vi "ObjectCacher(VariantInterface).vi"(8 "Enum(Get)":T1=enum."Get", 9 "type-postfix":string, 10 "Variant":variant, 11 "key":string[](array[string])) -> (1 "found/Replace":bool[](array[boolean]), 2 "names":string[](array[string]), 3 "values":variant[](array[variant]), 4 "cacher":variant)   [LabVIEW 2017]
uses:
  ObjectCacher-Operation.ctl
  <userlib>/_OpenG.lib/md5/md5.llb/MD5 Message Digest (Hexadecimal String)__ogtk.vi
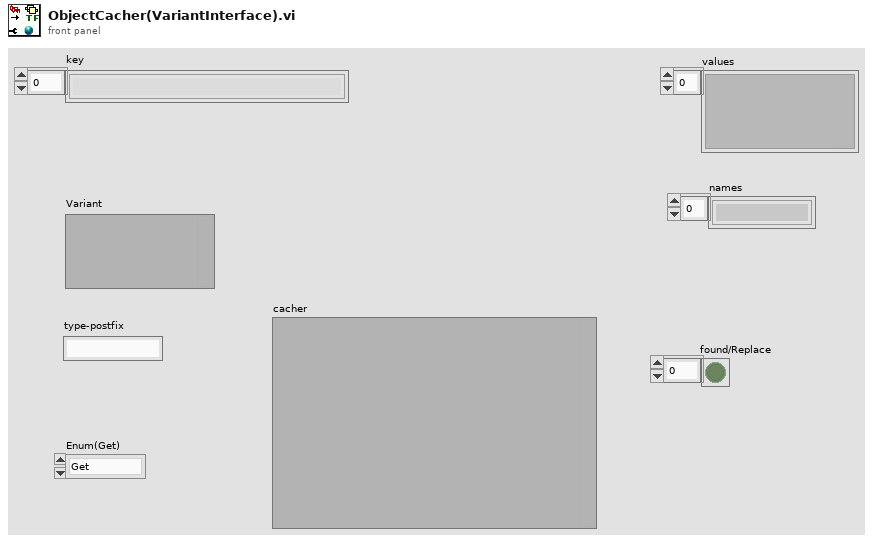
[diagram p1: front panel]
types:
  T1 = typedef "ObjectCacher-Operation.ctl" = enum16{"Reset", "Set", "Get", "Delete", "List", "<NONE>"}
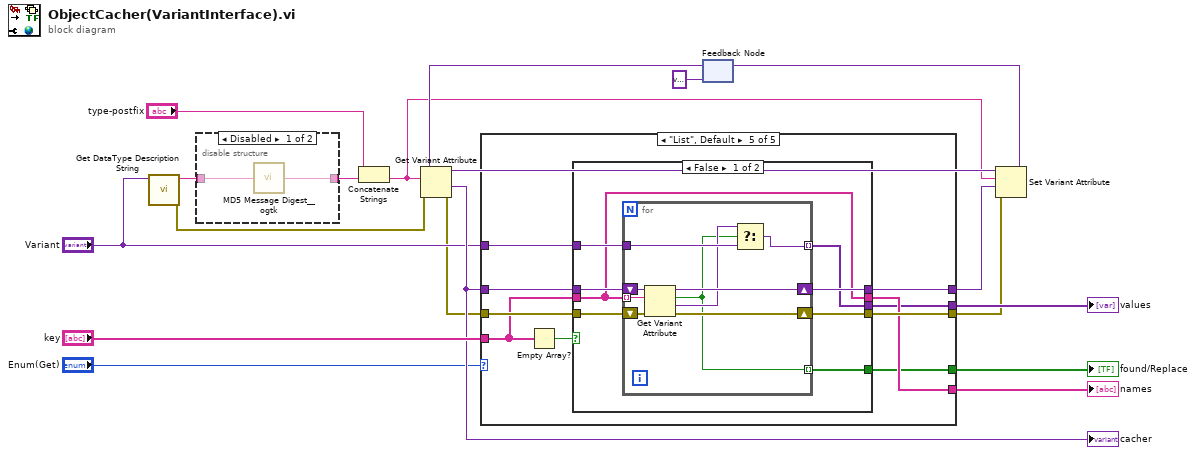
[diagram p0: block diagram]
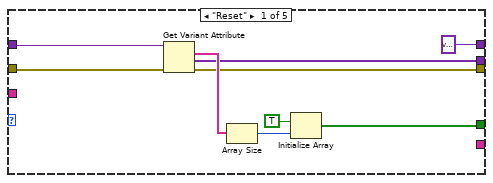
[diagram p2: hidden frame]
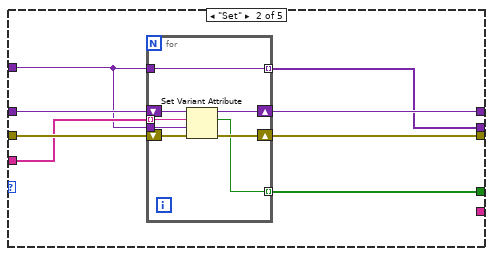
[diagram p3: hidden frame]
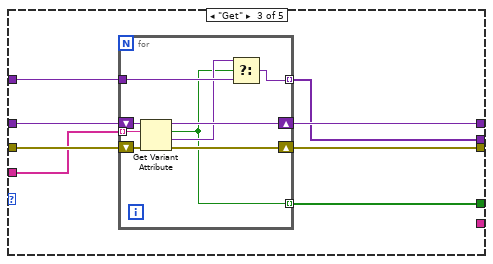
[diagram p4: hidden frame]
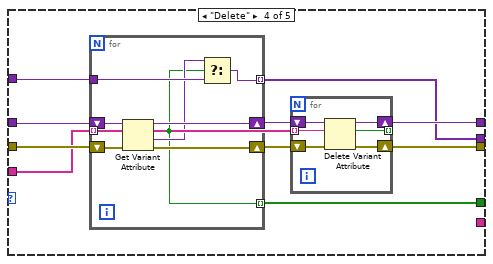
[diagram p5: hidden frame]
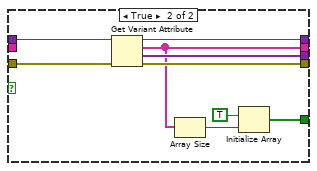
[diagram p6: hidden frame]
diagram:
  n1 = call "Get DataType Description String.vi"("Variant"="Variant") -> ("error out"=w1:errorcluster, "String"=w13:string)  [unwired: 9 in]
  n2 = disable-structure shown="Disabled" {
    disable-tunnel: w13 -> [w21 w22]
    disable-tunnel: [w20 w22] -> w12
    frame Disabled {
      n3 = call-poly <userlib>:"MD5 Message Digest__ogtk.vi"("Message"=w21) -> ("MD5 Message Digest"=w20:string)
    }
    frame Enabled {
    }
  }
  n4 = Concatenate Strings("type-postfix", w12) -> (w3:string)
  n5 = feedback #1(variant) -> (w16:variant)
  n6 = Get Variant Attribute(Variant=w16, name=w3, error in=w1) -> (duplicate Variant=w7:variant, value=w14:variant, error out=w5:errorcluster)  [unwired: 1 in, 1 out]
  "cacher" <- w14
  n7 = case shown="\"List\", Default" "Enum(Get)" {
    tunnel: [w24 w33 w49 w65 w94] -> w18
    tunnel: [variant w39 w55 w73 w96] -> w6
    tunnel: w5 -> [w27 w38 w54 w71 w99]
    tunnel: [w25 w37 w53 w74 w98] -> w4
    tunnel: w14 -> [w26 w36 w52 w72 w97]
    tunnel: "Variant" -> [_ w32 w50 w70 w91]
    tunnel: "key" -> [_ w35 w51 w69 w92]
    tunnel: [w23 w34 w48 w66 w90] -> w9
    tunnel: [_ _ _ _ w95] -> w8
    frame "Reset" {
      n8 = Get Variant Attribute(Variant=w26, error in=w27) -> (names=w30:string[], values=w24:variant[], error out=w25:errorcluster)  [unwired: 2 in, 1 out]
      n9 = Array Size(array=w30) -> (size(s)=w29:i32)
      n10 = Initialize Array(TRUE, w29) -> (w23:bool[])
    }
    frame "Set" {
      n11 = for {
        tunnel: w32 -> [w47]
        tunnel: w35 -> [w42] mode=indexing
        tunnel: [w41] -> w34 mode=indexing
        shift-right: [w44] -> w37
        shift-left: w38 -> [w45]
        shift-right: [w46] -> w39
        shift-left: w36 -> [w43]
        tunnel: [w40] -> w33 mode=indexing
        tunnel: w32 -> [w40]
        n12 = Set Variant Attribute(Variant=w43, name=w42, value=w47, error in=w45) -> (Variant out=w46:variant, replaced=w41:bool, error out=w44:errorcluster)
      }
    }
    frame "Get" {
      n13 = for {
        tunnel: w51 -> [w60] mode=indexing
        tunnel: [w56] -> w48 mode=indexing
        shift-right: [w62] -> w53
        shift-left: w54 -> [w63]
        shift-right: [w64] -> w55
        shift-left: w52 -> [w61]
        tunnel: w50 -> [w59]
        tunnel: [w57] -> w49 mode=indexing
        n14 = Get Variant Attribute(Variant=w61, name=w60, error in=w63) -> (duplicate Variant=w64:variant, found=w56:bool, value=w58:variant, error out=w62:errorcluster)  [unwired: 1 in]
        n15 = Select(t=w58, s=w56, f=w59) -> (s? t:f=w57:variant)
      }
    }
    frame "Delete" {
      n16 = for {
        tunnel: [w76] -> w66 mode=indexing
        shift-right: [w81] -> w67
        shift-left: w71 -> [w82]
        shift-right: [w83] -> w68
        shift-left: w72 -> [w80]
        tunnel: w70 -> [w79]
        tunnel: [w77] -> w65 mode=indexing
        tunnel: w69 -> [w75] mode=indexing
        n17 = Get Variant Attribute(Variant=w80, name=w75, error in=w82) -> (duplicate Variant=w83:variant, found=w76:bool, value=w78:variant, error out=w81:errorcluster)  [unwired: 1 in]
        n18 = Select(t=w78, s=w76, f=w79) -> (s? t:f=w77:variant)
      }
      n19 = for {
        tunnel: w69 -> [w86] mode=indexing
        tunnel: [w84] -> _ mode=indexing
        shift-right: [w88] -> w74
        shift-left: w67 -> [w89]
        shift-right: [w85] -> w73
        shift-left: w68 -> [w87]
        n20 = Delete Variant Attribute(4:w89, 6:w86, 7:w87) -> (0:w88:errorcluster, 2:w84:bool, 3:w85:variant)
      }
    }
    frame "List", Default {
      n21 = Empty Array?(array=w92) -> (empty?=w93:bool)
      n22 = case shown="False" w93 {
        tunnel: w99 -> [w106 w125]
        tunnel: [w104 w124] -> w98
        tunnel: w97 -> [w107 w123]
        tunnel: [w105 w122] -> w96
        tunnel: [w100 w119] -> w95
        tunnel: [w103 w121] -> w94
        tunnel: w92 -> [w100 _]
        tunnel: w91 -> [w102 _]
        tunnel: [w101 w120] -> w90
        frame False {
          n23 = for {
            tunnel: [w108] -> _ mode=indexing
            tunnel: [w109] -> w101 mode=indexing
            shift-right: [w114] -> w104
            shift-left: w106 -> [w115]
            shift-right: [w116] -> w105
            shift-left: w107 -> [w113]
            tunnel: w102 -> [w112]
            tunnel: [w110] -> w103 mode=indexing
            tunnel: w100 -> [w108] mode=indexing
            n24 = Get Variant Attribute(Variant=w113, name=w108, error in=w115) -> (duplicate Variant=w116:variant, found=w109:bool, value=w111:variant, error out=w114:errorcluster)  [unwired: 1 in]
            n25 = Select(t=w111, s=w109, f=w112) -> (s? t:f=w110:variant)
          }
        }
        frame True {
          n26 = Get Variant Attribute(Variant=w123, error in=w125) -> (duplicate Variant=w122:variant, names=w119:string[], values=w121:variant[], error out=w124:errorcluster)  [unwired: 2 in]
          n27 = Array Size(array=w119) -> (size(s)=w118:i32)
          n28 = Initialize Array(TRUE, w118) -> (w120:bool[])
        }
      }
    }
  }
  "values" <- w18
  "found/Replace" <- w9
  "names" <- w8
  n29 = Set Variant Attribute(Variant=w7, name=w3, value=w6, error in=w4) -> (Variant out=w15:variant)  [unwired: 2 out]
  n30 = feedback-in #1(w15) -> ()
